vi "get_average_laser_power.vi"(0 "Laser Power Q":T2, 1 "Cancel Notifier":T1, 2 "Averaging Time /s":u32, 11 "Error in":errorcluster) -> (4 "Laser Power Q Out":T2, 13 "Average Power / J":dbl, 15 "Error out":errorcluster)   [LabVIEW 2023]
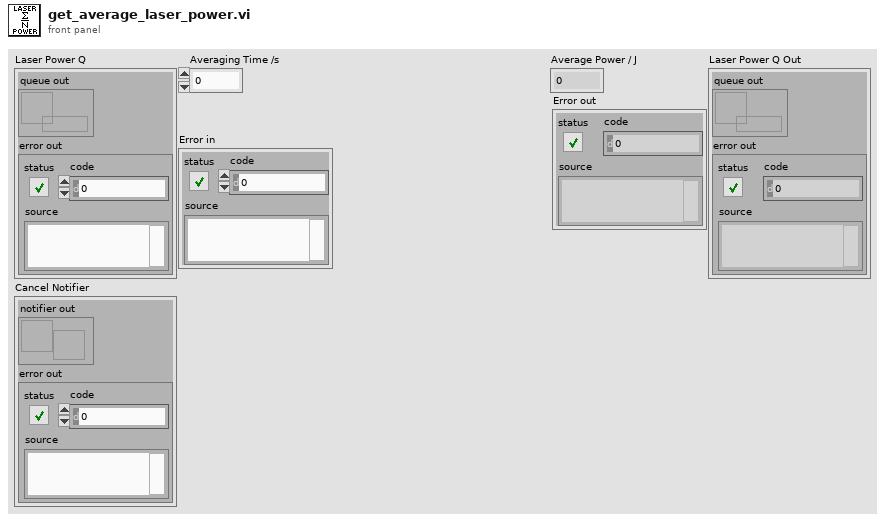
[diagram p1: front panel]
types:
  T1 = cluster{"notifier out":refnum<notifier>, "error out":errorcluster}
  T2 = cluster{"queue out":refnum<queue>, "error out":errorcluster}
  T3 = cluster{"Power Reading ":dbl, "T imestamp":dbl, "Status":i32}
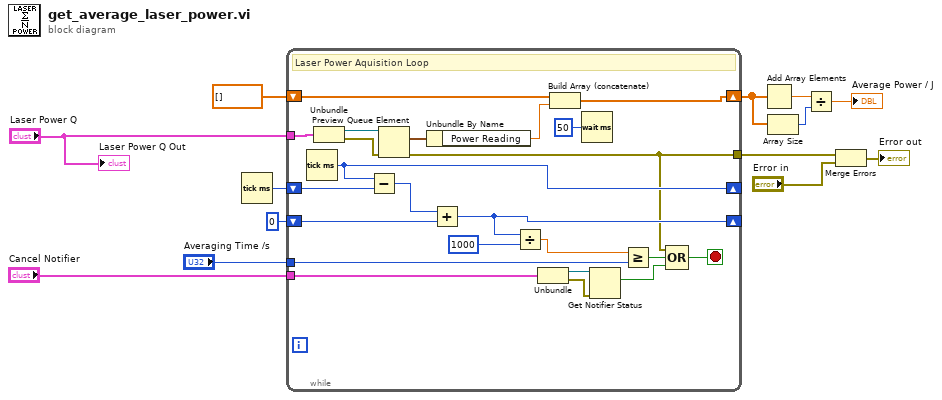
[diagram p0: block diagram]
diagram:
  n1 = Tick Count (ms)() -> (millisecond timer value=w11:u32)
  n2 = while {
    tunnel: "Laser Power Q" -> [w36]
    shift-right: [w29] -> w8
    shift-left: dbl[] [] -> [w31]
    shift-right: [w27] -> _
    shift-left: w11 -> [w28]
    shift-right: [w24] -> _
    shift-left: u32 0 -> [w25]
    tunnel: "Averaging Time /s" -> [w21]
    tunnel: [w19] -> w4
    tunnel: "Cancel Notifier" -> [w17]
    stop <- w18 stop-if-true
    # "Laser Power Aquisition Loop"
    n3 = Tick Count (ms)() -> (millisecond timer value=w27:u32)
    n4 = Unbundle(w36) -> ("queue out"=w35:refnum<queue>, "error out"=w34:errorcluster)
    n5 = Subtract(x=w27, y=w28) -> (x-y=w26:u32)
    n6 = Preview Queue Element(queue=w35, error in (no error)=w34) -> (element=w33:T3, error out=w19:errorcluster)  [unwired: 1 in, 2 out]
    n7 = Unbundle By Name(w33) -> ("Power Reading"=w32:dbl)
    n8 = Add(x=w26, y=w25) -> (x+y=w24:u32)
    n9 = Divide(x=w24, y=u32 1000) -> (x/y=w22:dbl)
    n10 = Unbundle(w17) -> ("notifier out"=w15:refnum<notifier>, "error out"=w14:errorcluster)
    n11 = Build Array (concatenate)(w31, w32) -> (w29:dbl[])
    n12 = Wait (ms)(milliseconds to wait=u32 50) -> ()  [unwired: 1 out]
    n13 = Get Notifier Status(notifier=w15, error in (no error)=w14) -> (current notification=w16:bool)  [unwired: 4 out]
    n14 = Greater Or Equal?(x=w22, y=w21) -> (x >= y?=w20:bool)
    n15 = Compound Arithmetic op=OR(w19, w20, w16) -> (w18:bool)
  }
  n16 = Add Array Elements(numeric array=w8) -> (sum=w9:dbl)
  n17 = Array Size(array=w8) -> (size(s)=w7:i32)
  n18 = Divide(x=w9, y=w7) -> (x/y=→"Average Power / J":dbl)
  n19 = Merge Errors(w4, "Error in") -> (→"Error out":errorcluster)
  "Laser Power Q Out" <- "Laser Power Q"
